vi "Disconnect.vi"(8 "error in (no error)":errorcluster, 11 "ESM303 in":refnum<class "ESM303.lvclass">) -> (0 "error out":errorcluster, 3 "ESM303 out":refnum<class "ESM303.lvclass">)   [LabVIEW 2018, in "ESM303.lvlib" / "ESM303.lvclass"]
uses:
  ESM303.lvclass
  builds/Force Test Stand.lvlibp/Force Test Stand.lvclass
  C:/Users/Ron.Dexter.LUMINARTECH/Desktop/builds/Force Test Stand.lvlibp/Force Test Stand.lvclass
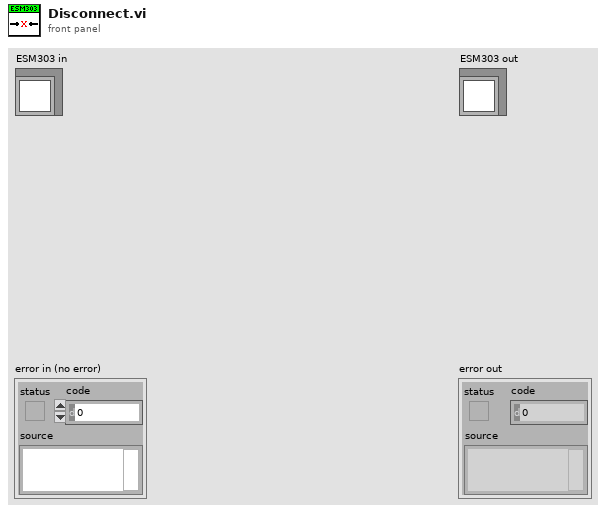
[diagram p1: front panel]
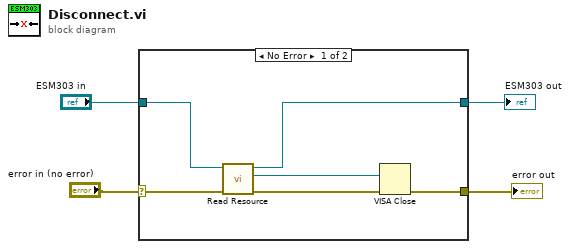
[diagram p0: block diagram]
diagram:
  n1 = case shown="No Error" "error in (no error)" {
    selector: "error in (no error)" -> [w10 w12]
    tunnel: [w6 w12] -> w3
    tunnel: [w8 w11] -> w2
    tunnel: "ESM303 in" -> [w9 w11]
    frame No Error {
      n2 = call "Read Resource.vi"("error in (no error)"=w10, "Force Test Stand in"=w9) -> ("error out"=w7:errorcluster, "Resource"=w5:refnum<visa-resource-name>, "Force Test Stand out"=w8:refnum<class "ESM303.lvclass">)  [unwired: 7 in]
      n3 = VISA Close(VISA resource name=w5, error in (no error)=w7) -> (error out=w6:errorcluster)
    }
    frame Error {
    }
  }
  "error out" <- w3
  "ESM303 out" <- w2
